vi "Meas Sequence Loop.vi"(8 "error in":errorcluster, 11 "meas session in":T1={"adc"={"niScope"={"channel cfg"=[], "sessions"=[], "multi cards"=FALSE, "channels"=0, "type"=enum."n/a", "memory [B/chn]"=0, "ext. clock [Hz]"=0.0, "samples count"=0, "use streaming"=FALSE, "proc setup"={"packet size [smpl]"=0, "current timeout [s]"=0.0, "blk2blk timeout [s]"=0.0, "event time"=timestamp(0 s since 1904-01-01), "temp sampl T [s]"=0.0, "data queue"=refnum, "stop notifier"=refnum, "proc ref"=refnum}, "sample width [B]"=0, "ranges [V]"=[], "trigger setup"={"coupling"=1, "level [V]"=0.0, "slope"=0, "mode"=enum."Immediate"}, "fs [Hz]"=0.0, "bitres [bit]"=0, "clock source"=enum."VAL_NO_SOURCE"}, "3458A"={"channels"=[], "sync unit"={"VISA"="", "type"=enum."Picotest U6200A"}, "awg unit"={"type"=enum."Agilent 331xxA to 332xxA", "VISA"="", "enable 10MHz ref"=FALSE, "cmi ckd2"={"VISA"="", "clock source"=enum."Auto", "manual ref clk"=FALSE, "ref clock [Hz]"=0.0}}, "sync mode"=enum."MASTER-SLAVE, MASTER clocked by TIMER", "streaming mode"=FALSE, "idn mode"=enum."Auto", "sampling mode"=enum."DCV", "Ts [s]"=0.0, "sample memory [B]"=0, "proc setup"={"channel id"=0, "packet size [smpl]"=0, "current timeout [s]"=0.0, "blk2blk timeout [s]"=0.0, "event time"=timestamp(0 s since 1904-01-01), "stop notifier"=refnum, "data queues"=[], "proc refs"=[], "bus semaphore"=refnum}, "sample size [B]"=0, "sample count"=0, "aux data"={"channel id"=0, "valid?"=[], "gain [V]"=[], "timestamp [s]"=[], "Ts [s]"=0.0, "abs timestamp"=timestamp(0 s since 1904-01-01), "t [deg C]"=[], "multiplex timestamp [s]"=-1.0, "only multiplex?"=FALSE, "multiplex smpl offset"=0}, "ranges [V]"=[], "aperture [s]"=0.0, "LEVEL trigger"={"edge"=enum."POS", "level [V]"=0.0, "coupling"=enum."DC"}, "trigger mode"=enum."AUTO", "measure temp.?"=FALSE, "disp mesages"=[], "shared bus?"=FALSE, "disable display?"=FALSE, "aper mode"=enum."Manual", "aper rules"=[], "multiplex"={"cycles"=0, "delay [s]"=0.0, "enabled"=FALSE, "overhead [s]"=1.0, "tot smpls"=0, "sub-rec"=0, "overhead [%]"=0.0}, "F8588 lpf"=enum."Off", "F8588 pll"=enum."Off", "F8588 couple"=enum."DC, auto"}, "dsdll"={"dsdll"={"dsdll path"=path "", "dsdll handle"=[], "output devices"=[], "capture devices"=[]}, "channels"=0, "device id"=0, "channel idns"=[], "proc setup"={"packet size [smpl]"=0, "current timeout [s]"=0.0, "blk2blk timeout [s]"=0.0, "event time"=timestamp(0 s since 1904-01-01), "data queue"=refnum, "stop notifier"=refnum, "proc ref"=refnum}, "samples count"=0, "fs [Hz]"=0.0}, "type"=enum."niScope", "channel idn str"=[], "aux instr idn str"=[], "modified?"=FALSE, "simadc"={"channels"=[], "range [V]"=0.0, "Ts step [s]"=0.0, "time [s]"=0.0, "fs [Hz]"=0.0, "count"=0, "smpl offset"=0, "set count"=0, "bit res"=0}, "force rst?"=FALSE, "exit mode"=enum."Immediate reset", "exit dly"=0.0, "exit tmr"=timestamp(0 s since 1904-01-01), "busy?"=FALSE, "accessed?"=FALSE, "multiplex"={"Type"=enum."Dummy", "gen com ssn"={"visa"="", "primary"=enum."None", "secondary"=enum."None", "channels"=[]}, "delay before [s]"=0.0, "delay post [s]"=0.0, "sequence"=[], "enabled"=FALSE, "ref timestamp [s]"=0.0, "idn string"="", "dev niScope"="", "niScope idx"=0}, "keysight dso"={"VISA"="", "channels"=[], "bw limit [Hz]"=0.0, "resolution"=enum."Auto", "trig noise reject"=enum."Normal", "N"=0, "trigger config"={"trigger source"=enum."Immediate", "level [V]"=0.0, "trigger slope"=enum."Negative"}, "fs [Hz]"=0.0, "timeout stop"=timestamp(0 s since 1904-01-01), "waiting for opc"=FALSE, "fetch offset [smpl]"=0, "abs timestamp"=timestamp(0 s since 1904-01-01), "ranges [V]"=[]}, "cdaq"={"mclk [Hz]"=12800000.0, "ADC task"="", "mclk reference"="", "fs [Hz]"=50000.0, "queue adc cmd"=refnum, "queue adc data"=refnum, "adc proc ref"=refnum, "channels"=[], "last channels"=[], "timeout"=timestamp(0 s since 1904-01-01), "N"=1000}}, "sequence"=[], "sequence setup"={"group setups"=[], "rec count"=0, "range mode"=enum."Keep defaults", "fs mode"=enum."Frequency", "rng even"=0.0, "rng odd"=0.0, "folder"=path "", "name base"="", "meas id"=0, "settle [s]"=0.0, "comment"="", "avg count"=0}, "golpi"=refnum, "processing setup"={"mode"=enum."Raw", "call after avgs?"=FALSE, "calculate?"=FALSE, "raw mode"={"command"="", "result mode"=enum."Display console output (only Octave)", "res variable"=""}, "QWTB"={"QWTB path"=path "", "alg filter path"="", "alg ids"=[], "alg parameters"=[], "parsed parameters"=[], "selected alg id"="", "selected unc mode"=enum."None", "qwtb mcc"=100, "qwtb timeout"=90, "qwtb covg"=95.0, "qwtb ofs"=0, "qwtb lim data"=0, "multicore"={"jobs folder"=path "", "cores"=0, "max jobs"=0, "mode"=enum."Singlecore"}, "unc once?"=FALSE, "qwtb tstemp"=enum."Enabled (default)", "octave reset"=FALSE, "exec mode"=enum."Single-core"}}, "corrections"={"transducers"={"channels"=[], "last path"=path ""}, "digitizer"={"last path"=path "", "channel paths"=[], "channel idns"=[], "correction name"="", "channel names"=[], "folders to copy"=[], "channel valid"=[], "correction path"=path "", "correction rel path"="", "rel folders to copy"=[]}}, "assist cfg"={"P"=0, "Q"=0, "rel shift"=0.0, "ref freq"=0.0, "min fs"=0.0, "max fs tol"=0.0, "min int"=0.0, "max int"=0.0, "max err"=0.0, "max timeout"=0.0}} {"corrections"."transducers"."channels"."Phase index" min=1 step=1; "adc"."cdaq"."last channels"."Channel id" min=0 step=1; "adc"."cdaq"."channels"."Channel id" min=0 step=1; "adc"."keysight dso"."bw limit [Hz]" format="%#_6p"; "adc"."keysight dso"."channels"."Offset [V]" min=0.0 format="%#_6p"; "adc"."keysight dso"."channels"."Range [Vpk]" min=0.0 format="%#_6p"; "adc"."keysight dso"."channels"."Channel" min=1; "adc"."3458A"."channels"."Range [Vpk]" min=0.0; "adc"."niScope"."trigger setup"."level [V]" format="%.2f"; "adc"."niScope"."trigger setup"."coupling" items=["AC"=0, "DC"=1, "HF Reject"=3, "LF Reject"=4, "AC Plus HF Reject"=1001]; "adc"."niScope"."channel cfg"."Range [Vpk]" min=0.0; "adc"."niScope"."channel cfg"."Channel" min=0}) -> (0 "error out":errorcluster, 3 "meas session out":T1={"adc"={"niScope"={"channel cfg"=[], "sessions"=[], "multi cards"=FALSE, "channels"=0, "type"=enum."n/a", "memory [B/chn]"=0, "ext. clock [Hz]"=0.0, "samples count"=0, "use streaming"=FALSE, "proc setup"={"packet size [smpl]"=0, "current timeout [s]"=0.0, "blk2blk timeout [s]"=0.0, "event time"=timestamp(0 s since 1904-01-01), "temp sampl T [s]"=0.0, "data queue"=refnum, "stop notifier"=refnum, "proc ref"=refnum}, "sample width [B]"=0, "ranges [V]"=[], "trigger setup"={"coupling"=1, "level [V]"=0.0, "slope"=0, "mode"=enum."Immediate"}, "fs [Hz]"=0.0, "bitres [bit]"=0, "clock source"=enum."VAL_NO_SOURCE"}, "3458A"={"channels"=[], "sync unit"={"VISA"="", "type"=enum."Picotest U6200A"}, "awg unit"={"type"=enum."Agilent 331xxA to 332xxA", "VISA"="", "enable 10MHz ref"=FALSE, "cmi ckd2"={"VISA"="", "clock source"=enum."Auto", "manual ref clk"=FALSE, "ref clock [Hz]"=0.0}}, "sync mode"=enum."MASTER-SLAVE, MASTER clocked by TIMER", "streaming mode"=FALSE, "idn mode"=enum."Auto", "sampling mode"=enum."DCV", "Ts [s]"=0.0, "sample memory [B]"=0, "proc setup"={"channel id"=0, "packet size [smpl]"=0, "current timeout [s]"=0.0, "blk2blk timeout [s]"=0.0, "event time"=timestamp(0 s since 1904-01-01), "stop notifier"=refnum, "data queues"=[], "proc refs"=[], "bus semaphore"=refnum}, "sample size [B]"=0, "sample count"=0, "aux data"={"channel id"=0, "valid?"=[], "gain [V]"=[], "timestamp [s]"=[], "Ts [s]"=0.0, "abs timestamp"=timestamp(0 s since 1904-01-01), "t [deg C]"=[], "multiplex timestamp [s]"=-1.0, "only multiplex?"=FALSE, "multiplex smpl offset"=0}, "ranges [V]"=[], "aperture [s]"=0.0, "LEVEL trigger"={"edge"=enum."POS", "level [V]"=0.0, "coupling"=enum."DC"}, "trigger mode"=enum."AUTO", "measure temp.?"=FALSE, "disp mesages"=[], "shared bus?"=FALSE, "disable display?"=FALSE, "aper mode"=enum."Manual", "aper rules"=[], "multiplex"={"cycles"=0, "delay [s]"=0.0, "enabled"=FALSE, "overhead [s]"=1.0, "tot smpls"=0, "sub-rec"=0, "overhead [%]"=0.0}, "F8588 lpf"=enum."Off", "F8588 pll"=enum."Off", "F8588 couple"=enum."DC, auto"}, "dsdll"={"dsdll"={"dsdll path"=path "", "dsdll handle"=[], "output devices"=[], "capture devices"=[]}, "channels"=0, "device id"=0, "channel idns"=[], "proc setup"={"packet size [smpl]"=0, "current timeout [s]"=0.0, "blk2blk timeout [s]"=0.0, "event time"=timestamp(0 s since 1904-01-01), "data queue"=refnum, "stop notifier"=refnum, "proc ref"=refnum}, "samples count"=0, "fs [Hz]"=0.0}, "type"=enum."niScope", "channel idn str"=[], "aux instr idn str"=[], "modified?"=FALSE, "simadc"={"channels"=[], "range [V]"=0.0, "Ts step [s]"=0.0, "time [s]"=0.0, "fs [Hz]"=0.0, "count"=0, "smpl offset"=0, "set count"=0, "bit res"=0}, "force rst?"=FALSE, "exit mode"=enum."Immediate reset", "exit dly"=0.0, "exit tmr"=timestamp(0 s since 1904-01-01), "busy?"=FALSE, "accessed?"=FALSE, "multiplex"={"Type"=enum."Dummy", "gen com ssn"={"visa"="", "primary"=enum."None", "secondary"=enum."None", "channels"=[]}, "delay before [s]"=0.0, "delay post [s]"=0.0, "sequence"=[], "enabled"=FALSE, "ref timestamp [s]"=0.0, "idn string"="", "dev niScope"="", "niScope idx"=0}, "keysight dso"={"VISA"="", "channels"=[], "bw limit [Hz]"=0.0, "resolution"=enum."Auto", "trig noise reject"=enum."Normal", "N"=0, "trigger config"={"trigger source"=enum."Immediate", "level [V]"=0.0, "trigger slope"=enum."Negative"}, "fs [Hz]"=0.0, "timeout stop"=timestamp(0 s since 1904-01-01), "waiting for opc"=FALSE, "fetch offset [smpl]"=0, "abs timestamp"=timestamp(0 s since 1904-01-01), "ranges [V]"=[]}, "cdaq"={"mclk [Hz]"=12800000.0, "ADC task"="", "mclk reference"="", "fs [Hz]"=50000.0, "queue adc cmd"=refnum, "queue adc data"=refnum, "adc proc ref"=refnum, "channels"=[], "last channels"=[], "timeout"=timestamp(0 s since 1904-01-01), "N"=1000}}, "sequence"=[], "sequence setup"={"group setups"=[], "rec count"=0, "range mode"=enum."Keep defaults", "fs mode"=enum."Frequency", "rng even"=0.0, "rng odd"=0.0, "folder"=path "", "name base"="", "meas id"=0, "settle [s]"=0.0, "comment"="", "avg count"=0}, "golpi"=refnum, "processing setup"={"mode"=enum."Raw", "call after avgs?"=FALSE, "calculate?"=FALSE, "raw mode"={"command"="", "result mode"=enum."Display console output (only Octave)", "res variable"=""}, "QWTB"={"QWTB path"=path "", "alg filter path"="", "alg ids"=[], "alg parameters"=[], "parsed parameters"=[], "selected alg id"="", "selected unc mode"=enum."None", "qwtb mcc"=100, "qwtb timeout"=90, "qwtb covg"=95.0, "qwtb ofs"=0, "qwtb lim data"=0, "multicore"={"jobs folder"=path "", "cores"=0, "max jobs"=0, "mode"=enum."Singlecore"}, "unc once?"=FALSE, "qwtb tstemp"=enum."Enabled (default)", "octave reset"=FALSE, "exec mode"=enum."Single-core"}}, "corrections"={"transducers"={"channels"=[], "last path"=path ""}, "digitizer"={"last path"=path "", "channel paths"=[], "channel idns"=[], "correction name"="", "channel names"=[], "folders to copy"=[], "channel valid"=[], "correction path"=path "", "correction rel path"="", "rel folders to copy"=[]}}, "assist cfg"={"P"=0, "Q"=0, "rel shift"=0.0, "ref freq"=0.0, "min fs"=0.0, "max fs tol"=0.0, "min int"=0.0, "max int"=0.0, "max err"=0.0, "max timeout"=0.0}} {"corrections"."transducers"."channels"."Phase index" min=1 step=1; "adc"."cdaq"."last channels"."Channel id" min=0 step=1; "adc"."cdaq"."channels"."Channel id" min=0 step=1; "adc"."keysight dso"."bw limit [Hz]" format="%#_6p"; "adc"."keysight dso"."channels"."Offset [V]" min=0.0 format="%#_6p"; "adc"."keysight dso"."channels"."Range [Vpk]" min=0.0 format="%#_6p"; "adc"."keysight dso"."channels"."Channel" min=1; "adc"."3458A"."channels"."Range [Vpk]" min=0.0; "adc"."niScope"."trigger setup"."level [V]" format="%.2f"; "adc"."niScope"."trigger setup"."coupling" items=["AC"=0, "DC"=1, "HF Reject"=3, "LF Reject"=4, "AC Plus HF Reject"=1001]; "adc"."niScope"."channel cfg"."Range [Vpk]" min=0.0; "adc"."niScope"."channel cfg"."Channel" min=0})   [LabVIEW 2013]
doc: "This VI initiates sampling of one record with current setup of ADC. It streams the sample data to MAT file of a given path (without extension). The VI also appends logged temperatures to the MAT file. It will return ADC auxiliary data which are valid only if flag 'valid?' in the cluster is True (that should happen all the time except when the sampling was aborted for whatever reason). The VI responds to global stop button called 'btn stop' - it will abort sampling when it is in True state."
uses:
  Meas Session.ctl
  adc/ADC Session.ctl
  drivers/niScope/niScope Session.ctl
  drivers/niScope/niScope Virtual Channel Config.ctl
  drivers/niScope/niScope Virtual Channel Mode.ctl
  drivers/niScope/niScope Virtual Channel Input Z.ctl
  drivers/niScope/niScope Virtual Channel Coupling.ctl
  drivers/niScope/niScope Type.ctl
  drivers/niScope/niScope Digitizing Process Options.ctl
  drivers/niScope/niScope Data Packet.ctl
  drivers/niScope/niScope Trigger Setup.ctl
  <instrlib>/niScope/Controls/niScope trigger coupling.ctl
  <instrlib>/niScope/Controls/niScope trigger slope.ctl
  drivers/niScope/niScope Reference Clock.ctl
  drivers/DMM/3458A Digitizer Session.ctl
  drivers/DMM/3458A Virtual Channel Config.ctl
  drivers/Counter/Counter Session.ctl
  drivers/Counter/Counter Type.ctl
  drivers/AWG/AWG Session.ctl
  drivers/AWG/AWG Type.ctl
  drivers/AWG/CMI Clock Divider v2/CMI ckd2 Session.ctl
  drivers/AWG/CMI Clock Divider v2/CMI ckd2 Source Mode.ctl
  drivers/DMM/3458A Sync Mode.ctl
  drivers/DMM/3458A Idn Mode.ctl
  drivers/DMM/3458A Digitizing Low Levels/Configure/Sampling Mode.ctl
  drivers/DMM/3458A Digitizing Process Options.ctl
  drivers/DMM/3458A Data Packet.ctl
  drivers/DMM/3458A Aux Record Data.ctl
  drivers/DMM/3458A Digitizing Low Levels/Configure/Level Setup.ctl
  drivers/DMM/3458A Digitizing Low Levels/Configure/First Sample Trigger.ctl
  drivers/DMM/3458A Aperture Selection Mode.ctl
  drivers/DMM/3458A Multiplexing Config.ctl
  drivers/Fluke 8588A/F8588A Low Pass Filter.ctl
  drivers/Fluke 8588A/F8588A Phase Lock.ctl
  drivers/Fluke 8588A/F8588A Coupling.ctl
  drivers/dsdll/DSDLL Session.ctl
  drivers/dsdll/dsdll.lvlibp/dsdll_instance.ctl
  drivers/dsdll/dsdll.lvlibp/dsdll_device_record.ctl
  drivers/dsdll/DSDLL Process Config.ctl
  drivers/dsdll/DSDLL Data Packet.ctl
  adc/ADC Type.ctl
  drivers/simulated_adc/SimAdc Config.ctl
  drivers/simulated_adc/SimAdc Channel Cfg.ctl
  adc/ADC On Close Action.ctl
  adc/Multiplexer/MPX Session.ctl
  adc/Multiplexer/MPX Type.ctl
  drivers/Multiplexers/Generic COM/GCOMM Session.ctl
  drivers/Multiplexers/Generic COM/GCOMM Signal.ctl
  drivers/Multiplexers/Generic COM/GCOMM Virtual Channel.ctl
  drivers/Multiplexers/Generic COM/GCOMM Logic State.ctl
  drivers/Agilent DSO 90000/Virtual Digitizer/KeDSO session.ctl
  drivers/Agilent DSO 90000/Virtual Digitizer/KeDSO Virtual Channel.ctl
  drivers/Agilent DSO 90000/Virtual Digitizer/KeDSO Trigger Setup.ctl
  drivers/Agilent DSO 90000/Virtual Digitizer/KeDSO Trigger Source.ctl
  drivers/cdaq/cDAQ Session.ctl
  drivers/cdaq/low_level_old/cdaq_anal_adc_command.ctl
  drivers/cdaq/low_level_old/cdaq_anal_adc_data.ctl
  drivers/cdaq/cDAQ Virtual Channel.ctl
  Meas Sequence Item.ctl
  Meas Sampling Configuration.ctl
  adc/ADC Trig Config.ctl
  adc/ADC Trig Mode Source.ctl
  adc/ADC Trig Coupling.ctl
  adc/ADC Trig Slope.ctl
  processing/QWTB/Meas Proc QWTB Algorithm Parameter Data.ctl
  Meas Sequence Configuration.ctl
  Meas Range Mode.ctl
  Meas Sampling Rate Mode.ctl
  octave/golpi/mpc/golpi_session_ref.ctl
  octave/golpi/mpc/golpi_session.ctl
  octave/golpi/GOLPI Library.lvlibp/Public/GOLPI reference Type Def.ctl
  octave/golpi/GOLPI Library.lvlibp/LV Process source distribution/Pipe Handle.ctl
  processing/Meas Process Config.ctl
  processing/Meas Process Mode.ctl
  processing/Meas Process Raw Config.ctl
  processing/Meas Process Raw Result Mode.ctl
  processing/QWTB/Meas Proc QWTB Setup.ctl
  processing/QWTB/Meas Proc QWTB Uncertainty Mode.ctl
  processing/QWTB/Meas Proc QWTB Multicore Setup.ctl
  processing/QWTB/Meas Proc QWTB Multicore Type.ctl
  processing/Meas Process Time Stamp Mode.ctl
  processing/QWTB/Meas Proc QWTB Exec Mode.ctl
  Corrections/Corr Setup.ctl
  Corrections/Corr Tranducer Item.ctl
  Corrections/Corr Digitizers.ctl
  Assist/Assist Panel Setup.ctl
  varilib/SGUI Assign Multiple Strings With Tags By Label.vi
  varilib/varilib.lvlib
  drivers/niScope/niScope Virtual Digitizer.lvlib
  drivers/DMM/3458A Virtual Digitizer.lvlib
  drivers/Counter/Counter.lvlib
  drivers/AWG/AWG.lvlib
  drivers/DMM/3458A Digitizing Low Levels/3458A Digitizing Low Levels.lvlib
  drivers/dsdll/dsdll.lvlibp
  drivers/dsdll/DSDLL Virtual Digitizer.lvlib
  octave/golpi/GOLPI Library.lvlibp/LV Process source distribution/LV Process library.lvlib
  octave/golpi/GOLPI Library.lvlibp
  octave/golpi/mpc/GOLPI Multi Process.lvlib
panel:
  out "error signal":bool
  # "ADC:"
  # "ADC:"
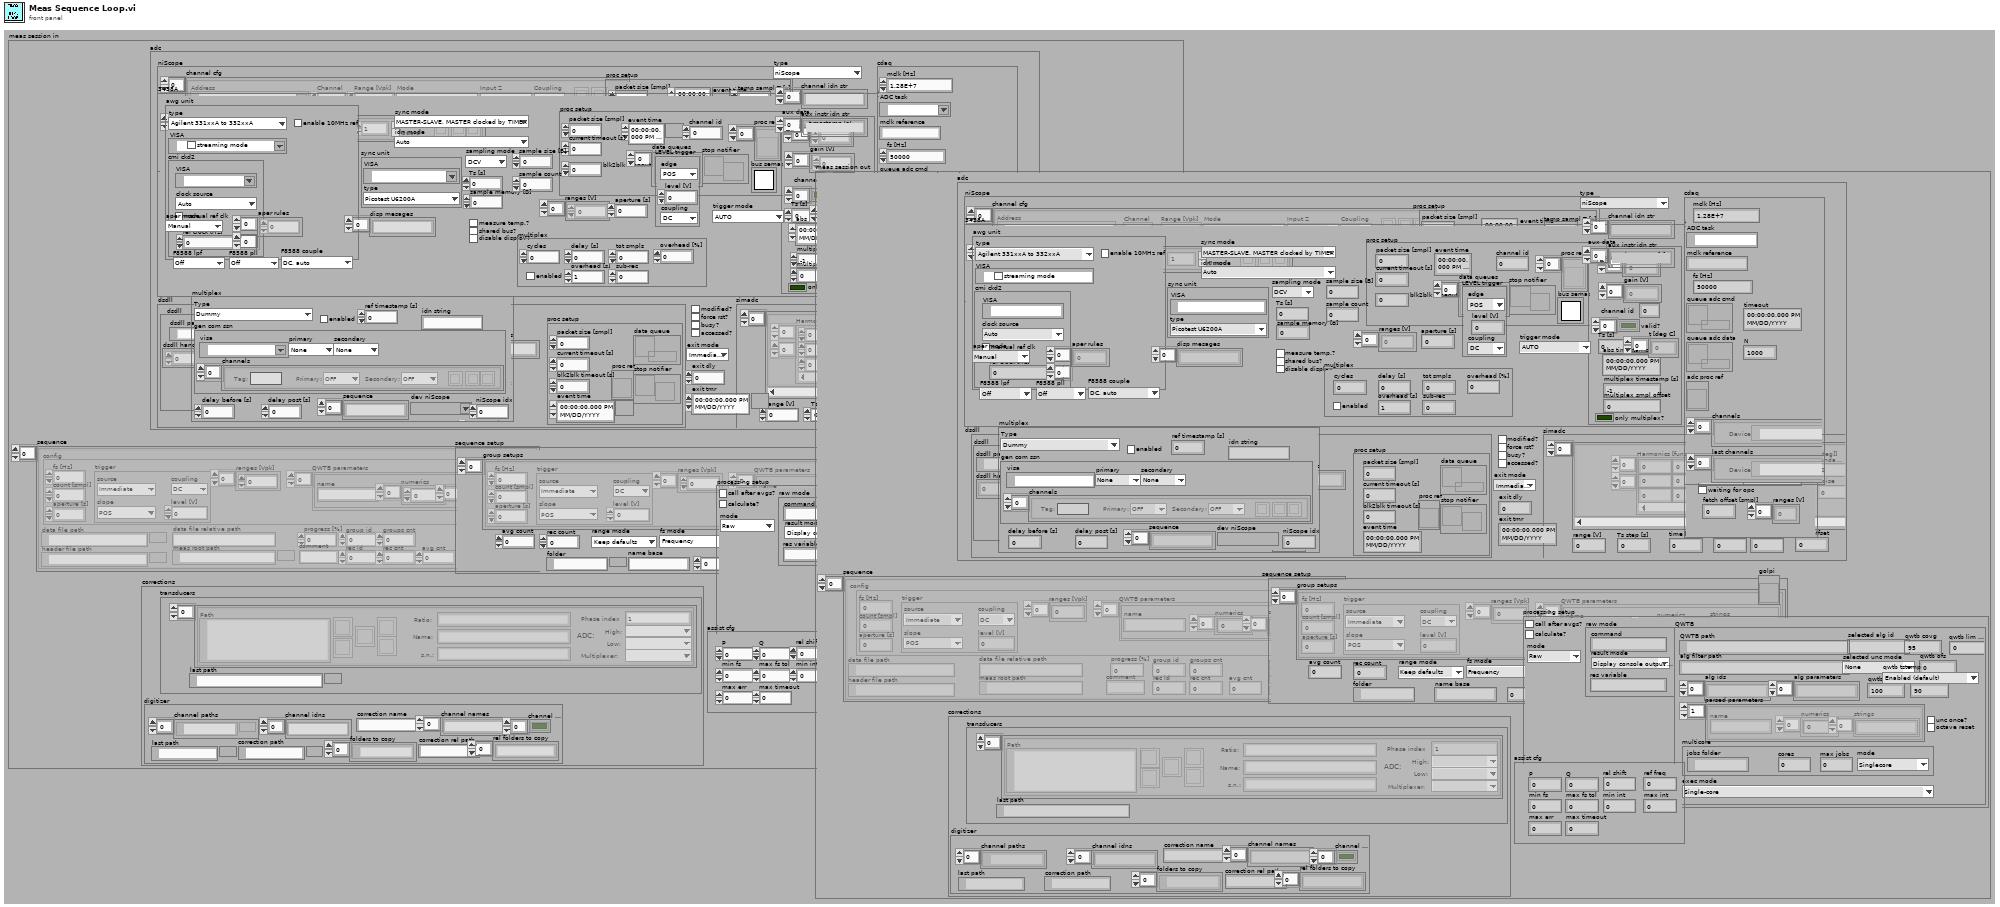
[diagram p1: front panel]
types:
  T1 = typedef "Meas Session.ctl" = cluster{"adc":T2, "sequence":T55[], "sequence setup":T62, "golpi":T65, "processing setup":T66, "corrections":T76, "assist cfg":T79}
  T2 = typedef "ADC Session.ctl" = cluster{"niScope":T3, "3458A":T14, "dsdll":T35, "type":T39, "channel idn str":string[], "aux instr idn str":string[], "modified?":bool, "simadc":T40, "force rst?":bool, "exit mode":T42, "exit dly":dbl, "exit tmr":timestamp, "busy?":bool, "accessed?":bool, "multiplex":T43, "keysight dso":T49, "cdaq":T53}
  T3 = typedef "niScope Virtual Digitizer.lvlib/niScope Session.ctl" = cluster{"channel cfg":T4[], "sessions":refnum<k20>[], "multi cards":bool, "channels":i32, "type":T8, "memory [B/chn]":i32, "ext. clock [Hz]":dbl, "samples count":i64, "use streaming":bool, "proc setup":T9, "sample width [B]":i32, "ranges [V]":dbl[], "trigger setup":T10, "fs [Hz]":dbl, "bitres [bit]":i32, "clock source":T13}
  T4 = typedef "niScope Virtual Digitizer.lvlib/niScope Virtual Channel Config.ctl" = cluster{"Address":refnum<k15>, "Channel":i32, "Mode":T5, "Input Z":T6, "Coupling":T7, "Range [Vpk]":dbl, "btn clr":bool, "btn up":bool, "btn down":bool}
  T5 = typedef "niScope Virtual Digitizer.lvlib/niScope Virtual Channel Mode.ctl" = enum16{"Single ended", "Unbal. differential", "Differential"}
  T6 = typedef "niScope Virtual Digitizer.lvlib/niScope Virtual Channel Input Z.ctl" = enum16{"1 MOhm", "50 Ohm"}
  T7 = typedef "niScope Virtual Digitizer.lvlib/niScope Virtual Channel Coupling.ctl" = enum16{"AC", "DC", "GND"}
  T8 = typedef "niScope Virtual Digitizer.lvlib/niScope Type.ctl" = enum16{"n/a", "5922"}
  T9 = typedef "niScope Virtual Digitizer.lvlib/niScope Digitizing Process Options.ctl" = cluster{"packet size [smpl]":i64, "current timeout [s]":dbl, "blk2blk timeout [s]":dbl, "event time":timestamp, "temp sampl T [s]":dbl, "data queue":refnum<queue>, "stop notifier":refnum<notifier>, "proc ref":refnum<vi>}
  T10 = typedef "niScope Virtual Digitizer.lvlib/niScope Trigger Setup.ctl" = cluster{"coupling":T11, "level [V]":dbl, "slope":T12, "mode":enum16{"Immediate", "External", "Level"}}
  T11 = typedef "niScope trigger coupling.ctl" = u16
  T12 = typedef "niScope trigger slope.ctl" = i32
  T13 = typedef "niScope Virtual Digitizer.lvlib/niScope Reference Clock.ctl" = enum16{"VAL_NO_SOURCE", "VAL_CLK_IN", "VAL_PXI_CLOCK", "VAL_EXTERNAL"}
  T14 = typedef "3458A Virtual Digitizer.lvlib/3458A Digitizer Session.ctl" = cluster{"channels":T15[], "sync unit":T16, "awg unit":T18, "sync mode":T22, "streaming mode":bool, "idn mode":T23, "sampling mode":T24, "Ts [s]":dbl, "sample memory [B]":i32, "proc setup":T25, "sample size [B]":i32, "sample count":i32, "aux data":T27, "ranges [V]":dbl[], "aperture [s]":dbl, "LEVEL trigger":T28, "trigger mode":T29, "measure temp.?":bool, "disp mesages":string[], "shared bus?":bool, "disable display?":bool, "aper mode":T30, "aper rules":dbl[][], "multiplex":T31, "F8588 lpf":T32, "F8588 pll":T33, "F8588 couple":T34}
  T15 = typedef "3458A Virtual Digitizer.lvlib/3458A Virtual Channel Config.ctl" = cluster{"VISA":refnum<visa-resource-name>, "Range [Vpk]":dbl, "btn clr":bool, "btn up":bool, "btn down":bool, "F8588":bool, "F8588 guard":bool}
  T16 = typedef "Counter.lvlib/Counter Session.ctl" = cluster{"VISA":refnum<visa-resource-name>, "type":T17}
  T17 = typedef "Counter.lvlib/Counter Type.ctl" = enum16{"Picotest U6200A", "dummy"}
  T18 = typedef "AWG.lvlib/AWG Session.ctl" = cluster{"type":T19, "VISA":refnum<visa-resource-name>, "enable 10MHz ref":bool, "cmi ckd2":T20}
  T19 = typedef "AWG.lvlib/AWG Type.ctl" = enum16{"Agilent 331xxA to 332xxA", "Agilent 335xxA to 336xxA", "Tektronix AFG3101C", "CMI Clock Divider v2", "dummy"}
  T20 = typedef "AWG.lvlib/CMI ckd2 Session.ctl" = cluster{"VISA":refnum<visa-resource-name>, "clock source":T21, "manual ref clk":bool, "ref clock [Hz]":dbl}
  T21 = typedef "AWG.lvlib/CMI ckd2 Source Mode.ctl" = enum16{"Auto", "LF clock", "HF clock", "Internal"}
  T22 = typedef "3458A Virtual Digitizer.lvlib/3458A Sync Mode.ctl" = enum16{"MASTER-SLAVE, MASTER clocked by TIMER", "MASTER-SLAVE, MASTER clocked by AWG", "ALL clocked by AWG", "MASTER-SLAVE, ALL clocked by TIMER", "ALL clocked by AWG with DFLL"}
  T23 = typedef "3458A Virtual Digitizer.lvlib/3458A Idn Mode.ctl" = enum16{"Auto", "Sequential (chn A, chn B, ...)", "From calibration string"}
  T24 = typedef "3458A Virtual Digitizer.lvlib/3458A Digitizing Low Levels.lvlib/Sampling Mode.ctl" = enum16{"DCV", "DSDC", "DSAC"}
  T25 = typedef "3458A Virtual Digitizer.lvlib/3458A Digitizing Process Options.ctl" = cluster{"channel id":i32, "packet size [smpl]":i32, "current timeout [s]":dbl, "blk2blk timeout [s]":dbl, "event time":timestamp, "stop notifier":refnum<notifier>, "data queues":refnum<queue>[], "proc refs":refnum<vi>[], "bus semaphore":T26}
  T26 = typedef "Semaphore RefNum" = refnum<k1>
  T27 = typedef "3458A Virtual Digitizer.lvlib/3458A Aux Record Data.ctl" = cluster{"channel id":i32, "valid?":bool[], "gain [V]":dbl[], "timestamp [s]":dbl[], "Ts [s]":dbl, "abs timestamp":timestamp, "t [deg C]":dbl[], "multiplex timestamp [s]":dbl, "only multiplex?":bool, "multiplex smpl offset":i64}
  T28 = typedef "3458A Virtual Digitizer.lvlib/3458A Digitizing Low Levels.lvlib/Level Setup.ctl" = cluster{"edge":enum16{"POS", "NEG"}, "level [V]":dbl, "coupling":enum16{"DC", "AC"}}
  T29 = typedef "3458A Virtual Digitizer.lvlib/3458A Digitizing Low Levels.lvlib/First Sample Trigger.ctl" = enum16{"AUTO", "EXT", "SYN", "SGL", "HOLD", "LEVEL"}
  T30 = typedef "3458A Virtual Digitizer.lvlib/3458A Aperture Selection Mode.ctl" = enum16{"Manual", "Maximum", "Table"}
  T31 = typedef "3458A Multiplexing Config.ctl" = cluster{"cycles":i32, "delay [s]":dbl, "enabled":bool, "overhead [s]":dbl, "tot smpls":i64, "sub-rec":i32, "overhead [%]":dbl}
  T32 = typedef "F8588A Low Pass Filter.ctl" = enum16{"Off", "100 kHz", "3 MHz"}
  T33 = typedef "F8588A Phase Lock.ctl" = enum16{"Off", "1 MHz", "10 MHz"}
  T34 = typedef "F8588A Coupling.ctl" = enum16{"AC, 1 MOhm", "AC, 10 MOhm", "DC, 1 MOhm", "DC, 10 MOhm", "DC, auto"}
  T35 = typedef "DSDLL Virtual Digitizer.lvlib/DSDLL Session.ctl" = cluster{"dsdll":T36, "channels":i32, "device id":i32, "channel idns":string[], "proc setup":T38, "samples count":i32, "fs [Hz]":dbl}
  T36 = typedef "dsdll.lvlibp/dsdll_instance.ctl" = cluster{"dsdll path":path, "dsdll handle":u8[], "output devices":T37[], "capture devices":T37[]}
  T37 = typedef "dsdll.lvlibp/dsdll_device_record.ctl" = cluster{"guid":u8[], "name":string}
  T38 = typedef "DSDLL Virtual Digitizer.lvlib/DSDLL Process Config.ctl" = cluster{"packet size [smpl]":i32, "current timeout [s]":dbl, "blk2blk timeout [s]":dbl, "event time":timestamp, "data queue":refnum<queue>, "stop notifier":refnum<notifier>, "proc ref":refnum<vi>}
  T39 = typedef "ADC Type.ctl" = enum16{"niScope", "3458A", "DirectSound DLL", "Keysight DSO", "cDAQ ADC", "dummy"}
  T40 = typedef "SimAdc Config.ctl" = cluster{"channels":T41[], "range [V]":dbl, "Ts step [s]":dbl, "time [s]":dbl, "fs [Hz]":dbl, "count":i64, "smpl offset":i64, "set count":i64, "bit res":i32}
  T41 = typedef "SimAdc Channel Cfg.ctl" = cluster{"harmonics":dbl[][], "btn clear":bool, "noise":dbl, "fundamental [Hz]":dbl}
  T42 = typedef "ADC On Close Action.ctl" = enum16{"Immediate reset", "Delayed reset"}
  T43 = typedef "MPX Session.ctl" = cluster{"Type":T44, "gen com ssn":T45, "delay before [s]":dbl, "delay post [s]":dbl, "sequence":string[], "enabled":bool, "ref timestamp [s]":dbl, "idn string":string, "dev niScope":refnum<k15>, "niScope idx":i32}
  T44 = typedef "MPX Type.ctl" = enum16{"Dummy", "Generic - COM port", "Generic - niScope PFI"}
  T45 = typedef "GCOMM Session.ctl" = cluster{"visa":refnum<visa-resource-name>, "primary":T46, "secondary":T46, "channels":T47[]}
  T46 = typedef "GCOMM Signal.ctl" = enum16{"None", "DTR", "RTS"}
  T47 = typedef "GCOMM Virtual Channel.ctl" = cluster{"Primary:":T48, "Secondary:":T48, "btn clr":bool, "btn up":bool, "btn down":bool, "Tag:":string}
  T48 = typedef "GCOMM Logic State.ctl" = enum16{"OFF", "ON"}
  T49 = typedef "KeDSO session.ctl" = cluster{"VISA":refnum<visa-resource-name>, "channels":T50[], "bw limit [Hz]":dbl, "resolution":enum16{"Auto", "Bits 9", "Bits 10", "Bits 11", "Bits 12"}, "trig noise reject":enum16{"Normal", "High Sensitivity"}, "N":i64, "trigger config":T51, "fs [Hz]":dbl, "timeout stop":timestamp, "waiting for opc":bool, "fetch offset [smpl]":i64, "abs timestamp":timestamp, "ranges [V]":dbl[]}
  T50 = typedef "KeDSO Virtual Channel.ctl" = cluster{"Channel":i32, "Range [Vpk]":dbl, "btn clr":bool, "btn up":bool, "btn down":bool, "Offset [V]":dbl, "Coupling":enum16{"DC", "DC50", "AC", "LFR1"}, "bw limit enab":bool}
  T51 = typedef "KeDSO Trigger Setup.ctl" = cluster{"trigger source":T52, "level [V]":dbl, "trigger slope":enum16{"Negative", "Positive", "Either"}}
  T52 = typedef "KeDSO Trigger Source.ctl" = enum16{"Immediate", "Level", "AUX"}
  T53 = typedef "cDAQ Session.ctl" = cluster{"mclk [Hz]":dbl, "ADC task":refnum<k21>, "mclk reference":string, "fs [Hz]":dbl, "queue adc cmd":refnum<queue>, "queue adc data":refnum<queue>, "adc proc ref":refnum<vi>, "channels":T54[], "last channels":T54[], "timeout":timestamp, "N":i32}
  T54 = typedef "cDAQ Virtual Channel.ctl" = cluster{"Device":tag, "Channel id":i32, "btn clr":bool, "btn up":bool, "btn down":bool}
  T55 = typedef "Meas Sequence Item.ctl" = cluster{"config":T56, "data file path":path, "header file path":path, "group id":i32, "rec id":i32, "group done?":bool, "adc modified?":bool, "source modified?":bool, "progress [%]":dbl, "groups cnt":i32, "rec cnt":i32, "data file relative path":string, "meas root path":path, "calculate?":bool, "comment":string, "avg cnt":i32}
  T56 = typedef "Meas Sampling Configuration.ctl" = cluster{"fs [Hz]":dbl, "count [smpl]":i64, "aperture [s]":dbl, "trigger":T57, "ranges [Vpk]":dbl[], "QWTB parameters":T61[]}
  T57 = typedef "ADC Trig Config.ctl" = cluster{"source":T58, "level [V]":dbl, "coupling":T59, "slope":T60}
  T58 = typedef "ADC Trig Mode Source.ctl" = enum16{"Immediate", "External", "Level"}
  T59 = typedef "ADC Trig Coupling.ctl" = enum16{"DC", "AC"}
  T60 = typedef "ADC Trig Slope.ctl" = enum16{"POS", "NEG"}
  T61 = typedef "Meas Proc QWTB Algorithm Parameter Data.ctl" = cluster{"name":string, "numerics":dbl[], "strings":string[]}
  T62 = typedef "Meas Sequence Configuration.ctl" = cluster{"group setups":T56[], "rec count":i32, "range mode":T63, "fs mode":T64, "rng even":dbl, "rng odd":dbl, "folder":path, "name base":string, "meas id":i32, "settle [s]":dbl, "comment":string, "avg count":i32}
  T63 = typedef "Meas Range Mode.ctl" = enum16{"Keep defaults", "Set All channels", "Set Odd and Even channels"}
  T64 = typedef "Meas Sampling Rate Mode.ctl" = enum16{"Frequency", "Period"}
  T65 = typedef "GOLPI Multi Process.lvlib/golpi_session_ref.ctl" = refnum<vi>
  T66 = typedef "Meas Process Config.ctl" = cluster{"mode":T67, "call after avgs?":bool, "calculate?":bool, "raw mode":T68, "QWTB":T70}
  T67 = typedef "Meas Process Mode.ctl" = enum16{"Raw", "QWTB"}
  T68 = typedef "Meas Process Raw Config.ctl" = cluster{"command":string, "result mode":T69, "res variable":string}
  T69 = typedef "Meas Process Raw Result Mode.ctl" = enum16{"Display console output (only Octave)", "Display string variable", "Display result file %respath%"}
  T70 = typedef "Meas Proc QWTB Setup.ctl" = cluster{"QWTB path":path, "alg filter path":string, "alg ids":string[], "alg parameters":string[], "parsed parameters":T61[], "selected alg id":string, "selected unc mode":T71, "qwtb mcc":i32, "qwtb timeout":i32, "qwtb covg":dbl, "qwtb ofs":i64, "qwtb lim data":i64, "multicore":T72, "unc once?":bool, "qwtb tstemp":T74, "octave reset":bool, "exec mode":T75}
  T71 = typedef "Meas Proc QWTB Uncertainty Mode.ctl" = enum16{"None", "GUF", "Monte Carlo"}
  T72 = typedef "Meas Proc QWTB Multicore Setup.ctl" = cluster{"jobs folder":path, "cores":i32, "max jobs":i32, "mode":T73}
  T73 = typedef "Meas Proc QWTB Multicore Type.ctl" = enum16{"Singlecore", "Multicore", "Multistation"}
  T74 = typedef "Meas Process Time Stamp Mode.ctl" = enum16{"Enabled (default)", "Disabled", "Relative to 1. record"}
  T75 = typedef "Meas Proc QWTB Exec Mode.ctl" = enum16{"Single-core", "Parallel Record Processing"}
  T76 = typedef "Corr Setup.ctl" = cluster{"transducers":cluster{"channels":T77[], "last path":path}, "digitizer":T78}
  T77 = typedef "Corr Tranducer Item.ctl" = cluster{"Path":path, "Ratio:":string, "Name:":string, "btn rem":bool, "btn up":bool, "btn down":bool, "s.n.:":string, "btn open":bool, "ratio o/i":dbl, "chn hi":u16, "chn lo":u16, "Phase index":i32, "btn edit":bool, "mpx chn":u16}
  T78 = typedef "Corr Digitizers.ctl" = cluster{"last path":path, "channel paths":path[], "channel idns":string[], "correction name":string, "channel names":string[], "folders to copy":path[], "channel valid":bool[], "correction path":path, "correction rel path":string, "rel folders to copy":string[]}
  T79 = typedef "Assist Panel Setup.ctl" = cluster{"P":i32, "Q":i32, "rel shift":dbl, "ref freq":dbl, "min fs":dbl, "max fs tol":dbl, "min int":dbl, "max int":dbl, "max err":dbl, "max timeout":dbl}
  T80 = typedef "ADC Aux Data.ctl" = cluster{"offset [V]":dbl[], "gain [V]":dbl[], "time stamp [s]":dbl[], "increment [s]":dbl, "T smpl":i64[], "T [deg C]":dbl[][], "valid?":bool, "abs timestamp":timestamp, "only multiplex?":bool, "multiplex smpl offset":i64, "multiplex timestamp [s]":dbl}
  T81 = typedef "MPX Record Segment Info.ctl" = cluster{"multiplex smpl offset":i64, "multiplex timestamp [s]":dbl}
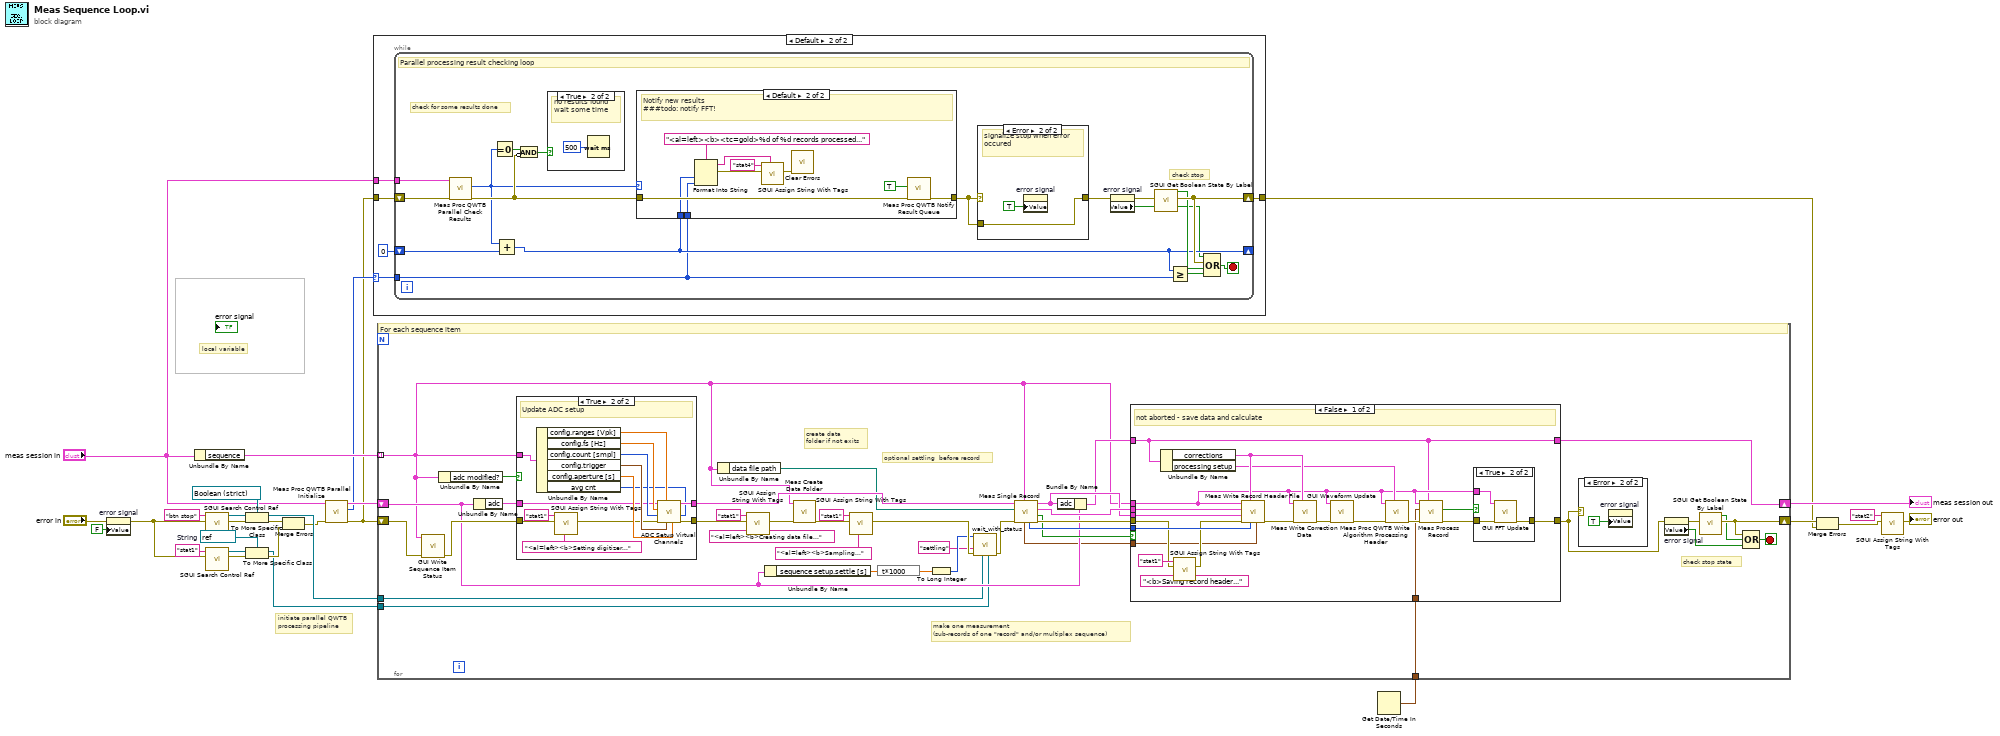
[diagram p0: block diagram]
diagram:
  w15 = refnum<vi> refnum  # String
  # "local variable"
  # "initiate parallel QWTB\nprocessing pipeline"
  n1 = property on="error signal" class="Bool (strict)"(error in="error in", "Value"=FALSE ("error signal")) -> (error out=w2:errorcluster)  [unwired: 1 in, 1 out]
  n2 = Unbundle By Name("meas session in") -> ("sequence"=w27:T55[])
  n3 = call "SGUI Search Control Ref.vi"("error in"=w2, "control label (empty)"="btn stop") -> ("error out"=w23:errorcluster, "control ref out"=w21:refnum<vi>)  [unwired: 7 in, 1 out]
  n4 = call "SGUI Search Control Ref.vi"("error in"=w2, "control label (empty)"="stat1") -> ("error out"=w20:errorcluster, "control ref out"=w17:refnum<vi>)  [unwired: 7 in, 1 out]
  n5 = To More Specific Class(target class=refnum<vi> refnum ("Boolean"), reference=w21, error in=w23) -> (specific class reference=w22:refnum<vi>, error out=w19:errorcluster)
  n6 = To More Specific Class(target class=w15, reference=w17, error in=w20) -> (specific class reference=w16:refnum<vi>, error out=w18:errorcluster)
  n7 = Merge Errors(w19, w18) -> (w11:errorcluster)
  n8 = call "Meas Proc QWTB Parallel Initialize.vi"("error in"=w11, "session"="meas session in") -> ("error out"=w8:errorcluster, "total results count"=w9:i16, "session out"=w10:T1)  [unwired: 7 in]
  n9 = case shown="Default" w9 {
    selector: w9 -> [_ w30]
    tunnel: w8 -> [w29 w34]
    tunnel: "meas session in" -> [_ w33]
    tunnel: [w29 w32] -> w5
    frame 0 {
    }
    frame Default {
      n10 = while {
        shift-right: [w44] -> w32
        shift-left: w34 -> [w51]
        tunnel: w33 -> [w50]
        shift-right: [w40] -> _
        shift-left: 0 -> [w49]
        tunnel: w30 -> [w39]
        stop <- w42 stop-if-true
        # "check stop"
        # "check for some results done"
        # "Parallel processing result checking loop"
        n11 = call "Meas Proc QWTB Parallel Check Results.vi"("error in"=w51, "session"=w50) -> ("error out"=w46:errorcluster, "done count"=w45:i32)  [unwired: 7 in, 1 out]
        n12 = Equal To 0?(x=w45) -> (x = 0?=w48:bool)
        n13 = Add(x=w45, y=w49) -> (x+y=w40:i32)
        n14 = Compound Arithmetic op=AND(w48, invert w46) -> (w47:bool)
        n15 = case shown="True" w47 {
          frame False {
          }
          frame True {
            # "no results found\nwait some time"
            n16 = Wait (ms)(milliseconds to wait=u32 500) -> ()  [unwired: 1 out]
          }
        }
        n17 = case shown="Default" w45 {
          tunnel: w46 -> [w55 w64]
          tunnel: [w55 w63] -> w38
          tunnel: w40 -> [_ w58]
          tunnel: w39 -> [_ w56]
          frame 0 {
          }
          frame Default {
            # "Notify new results\n###todo: notify FFT!"
            n18 = Format Into String(format string="<al=left><b><tc=gold>%d of %d records processed...", w58, w56) -> (resulting string=w60:string, error out=w61:errorcluster)  [unwired: 2 in]
            n19 = call-poly "SGUI Assign String With Tags.vi"("error in"=w61, "label(s) (empty)"="stat4", "string (empty)"=w60) -> ("error out"=w59:errorcluster)  [unwired: 7 in, 1 out]
            n20 = call <vilib>:"Clear Errors.vi"("error in (no error)"=w59) -> ()  [unwired: 6 in, 1 out]
            n21 = call "Meas Proc QWTB Notify Result Queue.vi"("error in"=w64, "new result? (False)"=TRUE) -> ("error out"=w63:errorcluster)  [unwired: 8 in, 1 out]
          }
        }
        n22 = case shown="Error" w38 {
          selector: w38 -> [w52 _]
          tunnel: [w52 w54] -> w37
          tunnel: w38 -> [_ w54]
          frame No Error {
          }
          frame Error {
            # "signalize stop when error occured"
            n23 = property on="error signal" class="Bool (strict)"("Value"=TRUE ("error signal")) -> ()  [unwired: 2 in, 2 out]
          }
        }
        n24 = property on="error signal" class="Bool (strict)"(error in=w37) -> (error out=w36:errorcluster, "Value"=w35:bool)  [unwired: 1 in, 1 out]
        n25 = call "SGUI Get Boolean State By Label.vi"("error in"=w36) -> ("error out"=w44:errorcluster, "binary state out"=w43:bool)  [unwired: 8 in, 1 out]
        n26 = Greater Or Equal?(x=w40, y=w39) -> (x >= y?=w41:bool)
        n27 = Compound Arithmetic op=OR(w35, w44, w43, w41) -> (w42:bool)
      }
    }
  }
  n28 = Get Date/Time In Seconds() -> (seconds since 1Jan1904=w12:timestamp)
  n29 = for {
    tunnel: w27 -> [w71] mode=indexing
    shift-right: [w95] -> w6
    shift-left: w8 -> [w82]
    shift-right: [w83] -> w28
    shift-left: w10 -> [w79]
    tunnel: w22 -> [w75]
    tunnel: w16 -> [w74]
    tunnel: w12 -> [w70]
    stop <- w96 stop-if-true
    # "optional settling  before record"
    # "create data\nfolder if not exits"
    # "check stop state"
    # "make one measurement\n(sub-records of one \"record\" and/or multiplex sequence)"
    # "For each sequence item"
    n30 = call "GUI Write Sequence Item Status.vi"("error in"=w82, "sequence item"=w71) -> ("error out"=w86:errorcluster)  [unwired: 8 in, 1 out]
    n31 = Unbundle By Name(w71) -> ("adc modified?"=w103:bool)
    n32 = Unbundle By Name(w79) -> ("adc"=w104:T2)
    n33 = case shown="True" w103 {
      tunnel: w86 -> [w132 w138]
      tunnel: w71 -> [_ w142]
      tunnel: w104 -> [w133 w141]
      tunnel: [w132 w140] -> w93
      tunnel: [w133 w139] -> w98
      frame False {
      }
      frame True {
        # "Update ADC setup"
        n34 = Unbundle By Name(w142) -> ("config.ranges [Vpk]"=w147:dbl[], "config.fs [Hz]"=w146:dbl, "config.count [smpl]"=w145:i64, "config.trigger"=w144:T57, "config.aperture [s]"=w143:dbl, "avg cnt"=w134:i32)
        n35 = call-poly "SGUI Assign String With Tags.vi"("error in"=w138, "label(s) (empty)"="stat1", "string (empty)"="<al=left><b>Setting digitizer...") -> ("error out"=w137:errorcluster)  [unwired: 7 in, 1 out]
        n36 = call "ADC Setup Virtual Channels.vi"("sub-records count"=w134, "apperture [s] (1.4 us)"=w143, "trigger (immediate)"=w144, "voltage ranges [Vpk] (empty: use global default)"=w147, "error in"=w137, "samples count (100)"=w145, "fs [Hz] (50k)"=w146, "adc session in"=w141) -> ("error out"=w140:errorcluster, "adc session out"=w139:T2)  [unwired: 2 in]
      }
    }
    n37 = Unbundle By Name(w71) -> ("data file path"=w85:path)
    n38 = call-poly "SGUI Assign String With Tags.vi"("error in"=w93, "label(s) (empty)"="stat1", "string (empty)"="<al=left><b>Creating data file...") -> ("error out"=w92:errorcluster)  [unwired: 7 in, 1 out]
    n39 = Unbundle By Name(w79) -> ("sequence setup.settle [s]"=w78:dbl)
    n40 = call "Meas Create Data Folder.vi"("error in"=w92, "sequence item"=w71) -> ("error out"=w89:errorcluster)  [unwired: 9 in]
    n41 = call-poly "SGUI Assign String With Tags.vi"("error in"=w89, "label(s) (empty)"="stat1", "string (empty)"="<al=left><b>Sampling...") -> ("error out"=w81:errorcluster)  [unwired: 7 in, 1 out]
    n42 = expression code="t*1000"(w78) -> (w77:dbl)
    n43 = To Long Integer(number=w77) -> (32bit integer=w76:i32)
    n44 = call "wait_with_status.vi"("stat ref"=w74, "stop ref"=w75, "error in"=w81, "comment"="settling", "ms to wait"=w76) -> ("error out"=w80:errorcluster)  [unwired: 6 in]
    n45 = call "Meas Single Record.vi"("sequence item"=w71, "error in"=w80, "binary data file path (no ext.)"=w85, "adc session in"=w98) -> ("error out"=w102:errorcluster, "aborted?"=w97:bool, "aux data"=w101:T80, "adc session out"=w100:T2, "acquired samples per channel"=w99:i64, "record segments info"=w72:T81[])  [unwired: 2 in]
    n46 = Bundle By Name(cluster=w79, "adc"=w100) -> (w84:T1)
    n47 = case shown="False" w97 {
      tunnel: w102 -> [w121 w131]
      tunnel: w101 -> [w125 _]
      tunnel: [w111 w131] -> w69
      tunnel: w71 -> [w110 _]
      tunnel: w100 -> [w124 _]
      tunnel: w99 -> [w123 _]
      tunnel: [w109 w130] -> w83
      tunnel: w84 -> [w109 w130]
      tunnel: w72 -> [w108 _]
      tunnel: w70 -> [w107 _]
      frame False {
        # "not aborted - save data and calculate"
        n48 = Unbundle By Name(w109) -> ("corrections"=w117:T76, "processing setup"=w113:T66)
        n49 = call-poly "SGUI Assign String With Tags.vi"("error in"=w121, "label(s) (empty)"="stat1", "string (empty)"="<b>Saving record header...") -> ("error out"=w120:errorcluster)  [unwired: 7 in, 1 out]
        n50 = call "Meas Write Record Header File.vi"("record segments info"=w108, "samples count"=w123, "corrections"=w117, "error in"=w120, "adc session"=w124, "aux data"=w125, "sequence item"=w110) -> ("error out"=w118:errorcluster)  [unwired: 4 in]
        n51 = call "Meas Write Correction Data.vi"("corrections"=w117, "error in"=w118, "sequence item"=w110) -> ("error out"=w116:errorcluster)  [unwired: 8 in]
        n52 = call "GUI Waveform Update.vi"("error in"=w116, "sequence item"=w110) -> ("error out"=w115:errorcluster)  [unwired: 9 in]
        n53 = call "Meas Proc QWTB Write Algorithm Processing Header.vi"("processing setup"=w113, "error in"=w115, "sequence item"=w110) -> ("error out"=w114:errorcluster)  [unwired: 8 in]
        n54 = call "Meas Process Record.vi"("session"=w109, "error in"=w114, "group time stamp"=w107, "sequence item"=w110) -> ("error out"=w112:errorcluster, "new result?"=w106:bool)  [unwired: 6 in]
        n55 = case shown="True" w106 {
          tunnel: w112 -> [w126 w129]
          tunnel: [w126 w128] -> w111
          tunnel: w110 -> [_ w127]
          frame False {
          }
          frame True {
            n56 = call "GUI FFT Update.vi"("error in"=w129, "sequence item"=w127) -> ("error out"=w128:errorcluster)  [unwired: 9 in]
          }
        }
      }
      frame True {
        # "aborted"
      }
    }
    n57 = case shown="Error" w69 {
      frame No Error {
      }
      frame Error {
        n58 = property on="error signal" class="Bool (strict)"("Value"=TRUE ("error signal")) -> ()  [unwired: 2 in, 2 out]
      }
    }
    n59 = property on="error signal" class="Bool (strict)"(error in=w69) -> (error out=w68:errorcluster, "Value"=w67:bool)  [unwired: 1 in, 1 out]
    n60 = call "SGUI Get Boolean State By Label.vi"("error in"=w68) -> ("error out"=w95:errorcluster, "binary state out"=w94:bool)  [unwired: 8 in, 1 out]
    n61 = Compound Arithmetic op=OR(w95, w94, w67) -> (w96:bool)
  }
  "meas session out" <- w28
  n62 = Merge Errors(w6, w5) -> (w4:errorcluster)
  n63 = call-poly "SGUI Assign String With Tags.vi"("error in"=w4, "label(s) (empty)"="stat2") -> ("error out"=→"error out":errorcluster)  [unwired: 8 in, 1 out]
